vi "Zamojski_Target_C_2.vi"   [LabVIEW 2020]
uses:
  <vilib>/Platform/TimedLoop/XDataNode/timing_clust.ctl
  <vilib>/Platform/TimedLoop/XDataNode/nitl_modes.ctl
  <vilib>/Platform/TimedLoop/XDataNode/wakeup.ctl
  <vilib>/platform/TimedLoop/XDataNode/XDataNode.xnode
  <vilib>/Platform/TimedLoop/XDataNode/XDNodeRunTimeDep.lvlib
types:
  T1 = typedef "XDNodeRunTimeDep.lvlib/timing_clust.ctl" = cluster{"Expected End [f-1]":u64, "Actual End [f-1]":u64, "Finished Late? [f-1]":bool, "Expected End [i-1]":u64, "Actual End [i-1]":u64, "Finished Late? [i-1]":bool, "Expected Start [i]":u64, "Actual Start [i]":u64, "Expected Start [f]":u64, "Actual Start [f]":u64, "Source Name":string, "Structure Name":string, "Period":i64, "Deadline":i64, "Offset":i64, "Start":i64, "Priority":i32, "Timeout":i32, "Mode":T2, "Wakeup Reason":T3, "Error":errorcluster, "Source Type":string, "Secondary Source Type":string, "Global End Time":u64, "Global Start Time":u64, "Frame Duration":u64, "Iteration Duration":u64, "Assigned CPU":i32, "I/O Scan Engine Mode":u32}
  T2 = typedef "XDNodeRunTimeDep.lvlib/nitl_modes.ctl" = enum32{"No Change", "Process missed periods, maintain original phase", "Discard missed periods, maintain original phase", "Process missed periods, ignore original phase", "Discard missed periods, ignore original phase"}
  T3 = typedef "XDNodeRunTimeDep.lvlib/wakeup.ctl" = enum32{"Normal", "Aborted", "Asynchronous wakeup", "Timing source error", "Timed loop error", "Timeout"}
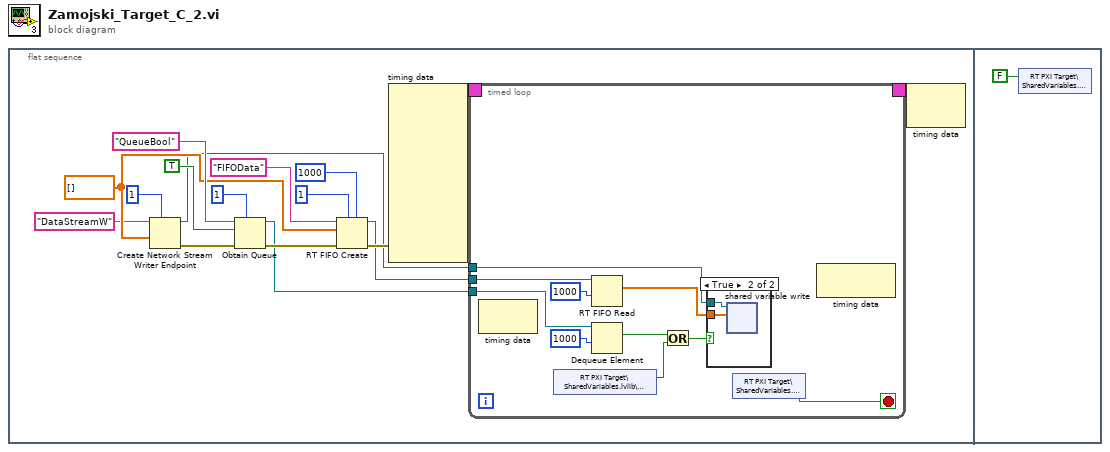
[diagram p0: block diagram]
diagram:
  n1 = flat-sequence {
    frame #0 {
      w5 = dbl[] []
      n2 = Create Network Stream Writer Endpoint(7:1 ("writer buffer size"), 9:w5, 11:"DataStreamW" ("writer name")) -> (0:w7:errorcluster, 3:w3:refnum<k21>)  [unwired: 4 in]
      n3 = Obtain Queue(max queue size (-1, unlimited)=1, name (unnamed)="QueueBool", element data type=TRUE, error in (no error)=w7) -> (queue out=w1:refnum<queue>, error out=w9:errorcluster)  [unwired: 1 in, 1 out]
      n4 = RT FIFO Create(0:"FIFOData" ("name (unnamed)"), 1:w5, 3:w9, 4:u32 1 ("size (10)"), 6:u32 1000 ("elements in array (1)")) -> (8:w2:refnum<k33>, 11:w8:errorcluster)  [unwired: 3 in, 1 out]
      n5 = node-c288(w8) -> (w17:T1)  [unwired: 9 in]
      n6 = timed-loop {
        timing: w17 -> [_]
        timing-out: [_] -> w16
        tunnel: w3 -> [w20]
        tunnel: w2 -> [w27]
        tunnel: w1 -> [w26]
        stop <- w18 stop-if-true
        n7 = node-c288() -> ()  [unwired: 1 in, 1 out]
        n8 = shared-variable "RT PXI Target\\SharedVariables.lvlib\\SignalSend"() -> (w23:bool)  [unwired: 1 in, 1 out]
        n9 = RT FIFO Read(0:w27, 2:1000 ("timeout ms (-1)")) -> (9:w19:dbl[])  [unwired: 2 in, 4 out]
        n10 = Dequeue Element(queue=w26, timeout in ms (-1)=1000) -> (element=w22:bool)  [unwired: 1 in, 3 out]
        n11 = Or(x=w22, y=w23) -> (x .or. y?=w24:bool)
        n12 = case shown="True" w24 {
          tunnel: w20 -> [_ w29]
          tunnel: w19 -> [_ w28]
          frame False {
          }
          frame True {
            n13 = shared-variable-write(w29, w28) -> ()  [unwired: 2 in, 3 out]
          }
        }
        n14 = shared-variable "RT PXI Target\\SharedVariables.lvlib\\STOP"() -> (w18:bool)  [unwired: 1 in, 1 out]
        n15 = node-c288() -> ()  [unwired: 1 in, 1 out]
      }
      n16 = node-c288(w16) -> ()  [unwired: 1 out]
    }
    frame #1 {
      n17 = shared-variable "RT PXI Target\\SharedVariables.lvlib\\STOP"(FALSE ("STOP")) -> ()  [unwired: 1 in, 1 out]
    }
  }
